vi "Profile not found--error.vi"(11 "Name":string) -> (0 "error out":errorcluster)   [LabVIEW 2025]
doc: "Indicates that the profile specified by the user does not exist."
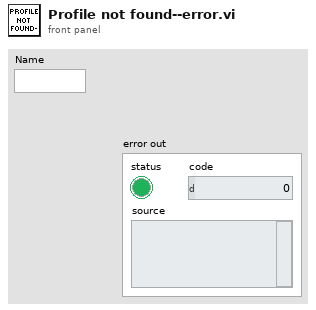
[diagram p1: front panel]
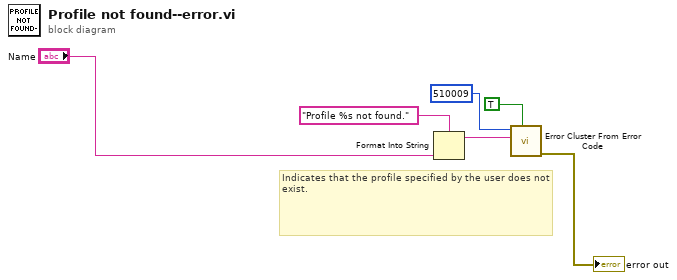
[diagram p0: block diagram]
diagram:
  # "Indicates that the profile specified by the user does not exist."
  n1 = Format Into String(format string="Profile %s not found." ("error message (\"\")"), "Name") -> (resulting string=w1:string)  [unwired: 2 in, 1 out]
  n2 = call <vilib>:"Error Cluster From Error Code.vi"("show call chain? (False)"=TRUE, "error message (\"\")"=w1, "error code (0)"=510009) -> ("error out"=→"error out":errorcluster)  [unwired: 6 in]
